vi "Display Feature Preview.vi"(7 "UI References":T1, 8 "error in (no error)":errorcluster, 10 "Features":string[][](array[string])) -> (0 "error out":errorcluster)   [LabVIEW 2024]
uses:
  Controls/RVHR - UI Refs.ctl
  <vilib>/picture/picture.llb/Draw True-Color Pixmap.vi
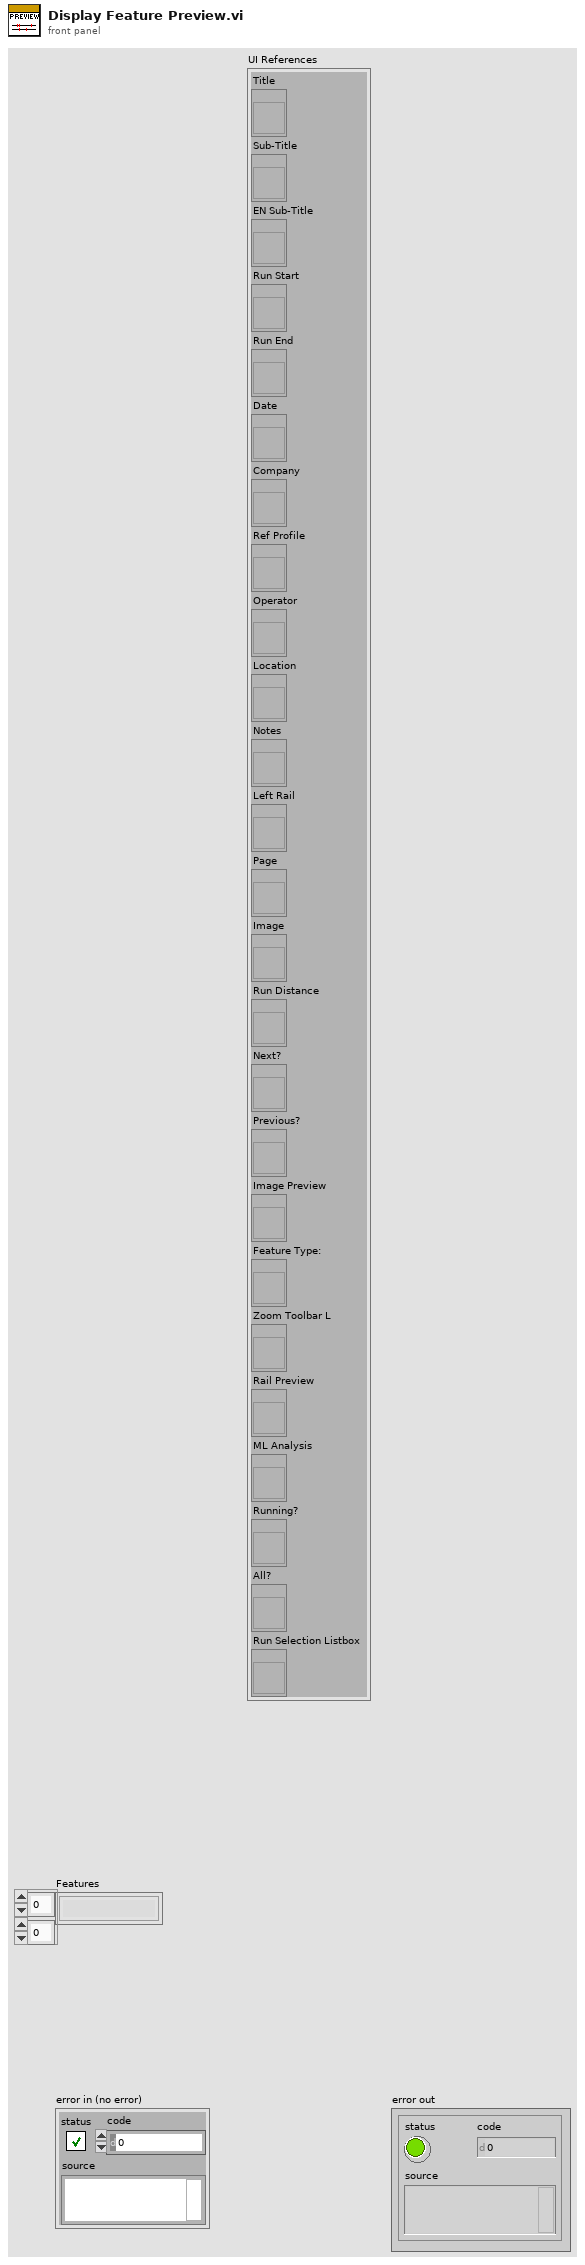
[diagram p1: front panel]
types:
  T1 = typedef "RVHR - UI Refs.ctl" = cluster{"Title":refnum<vi>, "Sub-Title":refnum<vi>, "EN Sub-Title":refnum<vi>, "Run Start":refnum<vi>, "Run End":refnum<vi>, "Date":refnum<vi>, "Company":refnum<vi>, "Ref Profile":refnum<vi>, "Operator":refnum<vi>, "Location":refnum<vi>, "Notes":refnum<vi>, "Left Rail":refnum<vi>, "Page":refnum<vi>, "Image":refnum<vi>, "Run Distance":refnum<vi>, "Next?":refnum<vi>, "Previous?":refnum<vi>, "Image Preview":refnum<vi>, "Feature Type:":refnum<vi>, "Zoom Toolbar L":refnum<vi>, "Rail Preview":refnum<vi>, "ML Analysis":refnum<vi>, "Running?":refnum<vi>, "All?":refnum<vi>, "Run Selection Listbox":refnum<vi>}
  T2 = typedef "LVBoundsTypeDef.ctl" = cluster{"Width":u32, "Height":u32}
  T3 = cluster{"[0]":i32, "[1]":i32, "[2]":i32, "[3]":i32}
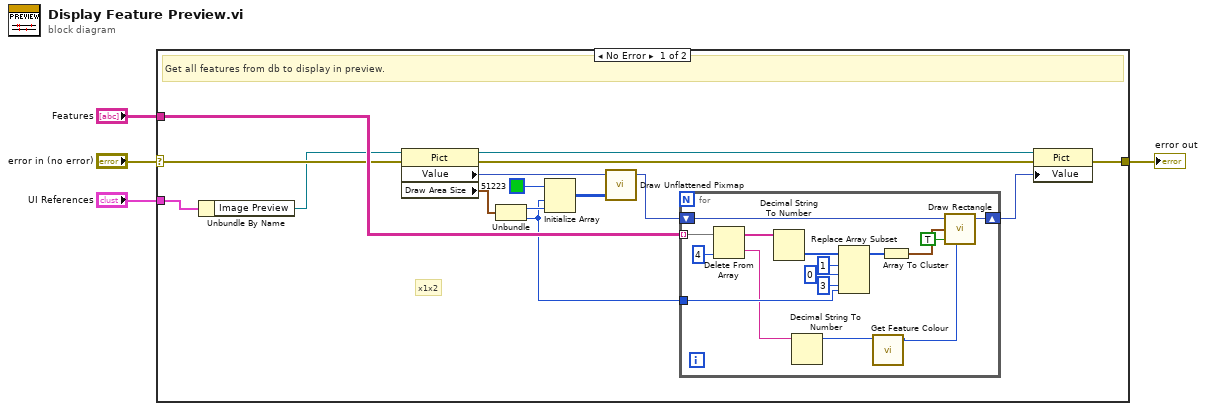
[diagram p0: block diagram]
diagram:
  n1 = case shown="No Error" "error in (no error)" {
    selector: "error in (no error)" -> [w17 w36]
    tunnel: [w12 w36] -> w3
    tunnel: "UI References" -> [w19 _]
    tunnel: "Features" -> [w18 _]
    frame No Error {
      # "x1x2"
      # "Get all features from db to display in preview."
      n2 = Unbundle By Name(w19) -> ("Image Preview"=w14:refnum<vi>)
      n3 = property class="Pict"(reference=w14, error in=w17) -> (reference out=w16:refnum<vi>, error out=w13:errorcluster, "Value"=w10:picture, "Draw Area Size"=w11:T2)
      n4 = Unbundle(w11) -> ("Width"=w8:u32, "Height"=w6:u32)
      n5 = Initialize Array(u32 51223 ("color(black)"), w6, w8) -> (w7:u32[][])
      n6 = call-poly <vilib>:"Draw Unflattened Pixmap.vi"("picture"=w10, "data (RGB format)"=w7) -> ("new picture"=w9:picture)  [unwired: 7 in]
      n7 = for {
        tunnel: w18 -> [w35] mode=indexing
        shift-right: [w30] -> w15
        shift-left: w9 -> [w31]
        tunnel: w6 -> [w24]
        n8 = Delete From Array(array=w35, index=4) -> (deleted portion=w21:string, array with subset deleted=w33:string[])  [unwired: 1 in]
        n9 = Decimal String To Number(string=w33) -> (number=w29:i32[])  [unwired: 2 in, 1 out]
        n10 = Decimal String To Number(string=w21) -> (number=w20:i32)  [unwired: 2 in, 1 out]
        n11 = Replace Array Subset(array=w29, new element #1=0 ("new element/subarray"), index #1=1 ("index"), new element #2=w24, index #2=3 ("index")) -> (w28:i32[])
        n12 = call "Get Feature Colour.vi"("Feature Type"=w20) -> ("color"=w22:u32)  [unwired: 10 in]
        n13 = Array To Cluster(array=w28) -> (cluster=w32:T3)
        n14 = call <vilib>:"Draw Rectangle.vi"("picture"=w31, "rect"=w32, "fill?(F)"=TRUE, "color(black)"=w22) -> ("new picture"=w30:picture)  [unwired: 5 in]
      }
      n15 = property class="Pict"(reference=w16, error in=w13, "Value"=w15) -> (error out=w12:errorcluster)  [unwired: 1 out]
    }
    frame Error {
    }
  }
  "error out" <- w3
